vi "S2C_M2p5942_Proc_Acquire.vi"(7 "Command":string, 8 "Error In":errorcluster, 10 "Stop?":bool, 11 "Data":T1) -> (0 "Error Out":errorcluster)   [LabVIEW 2024]
uses:
  S2C_M2p5942_Proc_Globals.vi
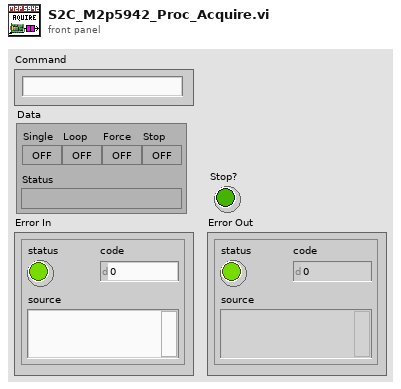
[diagram p1: front panel]
types:
  T1 = cluster{"Single":bool, "Loop":bool, "Force":bool, "Status":string, "Stop":bool}
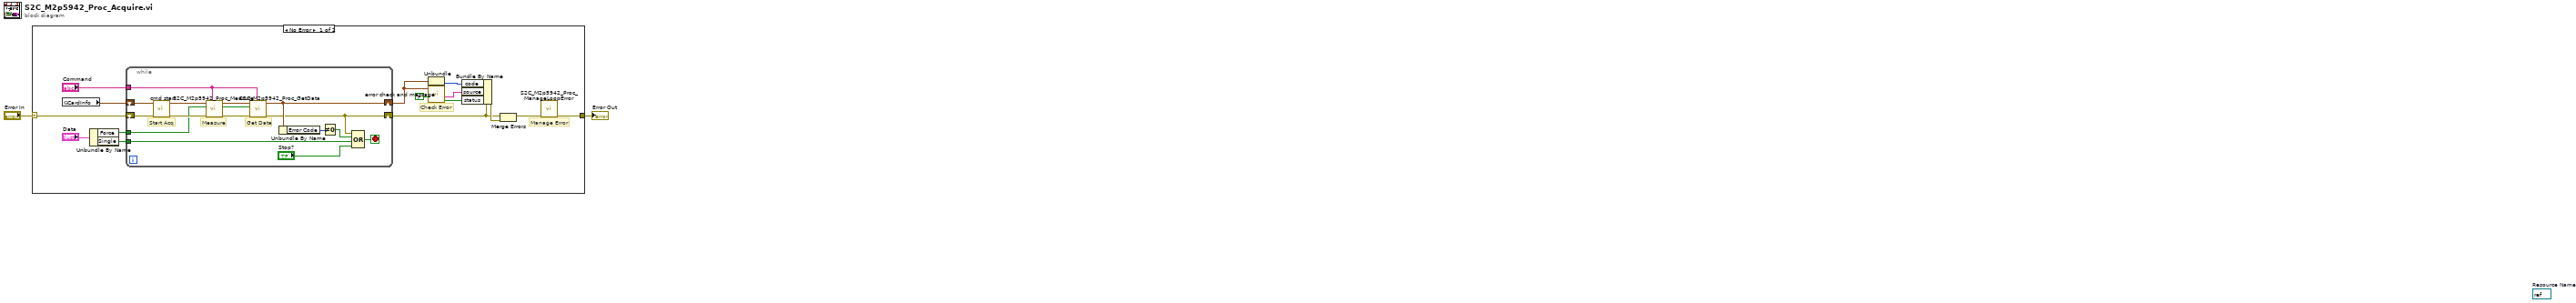
[diagram p0: block diagram]
diagram:
  (unwired) refnum<visa-resource-name> refnum  # Resource Name
  n1 = case shown="No Error" "Error In" {
    selector: "Error In" -> [w3 w33]
    tunnel: [w5 w33] -> w1
    frame No Error {
      # "Manage Error"
      # "Check Error"
      n2 = global read "S2C_M2p5942_Proc_Globals.vi" "CardInfo"() -> (w16:cluster{"Card Handle":u64, "Error Code":u32})
      n3 = Unbundle By Name("Data") -> ("Force"=w15:bool, "Single"=w14:bool)
      n4 = while {
        shift-right: [w20] -> w8
        shift-left: w3 -> [w32]
        tunnel: "Command" -> [w28]
        shift-right: [w24] -> w7
        shift-left: w16 -> [w27]
        tunnel: w15 -> [w25]
        tunnel: w14 -> [w23]
        stop <- w19 stop-if-true
        # "Start Acq"
        # "Get Data"
        # "Measure"
        n5 = call "cmd start.vi"("Card Info In"=w27) -> ("Card Info Out"=w26:cluster{"Card Handle":u64, "Error Code":u32})  [unwired: 6 in]
        n6 = call "S2C_M2p5942_Proc_Measure.vi"("Command"=w28, "Error In"=w32, "Force Trigger?"=w25, "Card In"=w26) -> ("Error Out"=w31:errorcluster, "Ready?"=w29:bool, "Card Out"=w30:cluster{"Card Handle":u64, "Error Code":u32})  [unwired: 5 in]
        n7 = call "S2C_M2p5942_Proc_GetData.vi"("Command"=w28, "Error In"=w31, "Ready?"=w29, "Card In"=w30) -> ("Error Out"=w20:errorcluster, "Card Out"=w24:cluster{"Card Handle":u64, "Error Code":u32})  [unwired: 6 in]
        n8 = Unbundle By Name(w24) -> ("Error Code"=w22:u32)
        n9 = Not Equal To 0?(x=w22) -> (x != 0?=w21:bool)
        n10 = Compound Arithmetic op=OR(w20, w21, w23, "Stop?") -> (w19:bool)
      }
      n11 = Unbundle(w7) -> ("Error Code"=w11:u32)  [unwired: 1 out]
      n12 = call "error check and message.vi"("Display Message (true)"=FALSE, "Card Info In"=w7) -> ("Error occurred"=w9:bool, "Error Message"=w10:string)  [unwired: 3 in, 1 out]
      n13 = Bundle By Name(cluster=w8, "code"=w11, "source"=w10, "status"=w9) -> (w13:errorcluster)
      n14 = Merge Errors(w8, w13) -> (w4:errorcluster)
      n15 = call "S2C_M2p5942_Proc_ManageLoopError.vi"("Error In"=w4) -> ("Error Out"=w5:errorcluster)  [unwired: 10 in]
    }
    frame Error {
    }
  }
  "Error Out" <- w1
